vi "Listen.vi"() -> ()   [LabVIEW 2017]
uses:
  WebSocket.lvclass
panel:
  out "trimmed string":string
  out "element":string
  out "Headers":variant=variant("Accept-Encoding"=variant(string "gzip, deflate, br"), "Accept-Language"=variant(string "en-US,en;q=0.9"), "Cache-Control"=variant(string "no-cache"), "Connection"=variant(string "Upgrade"), "Host"=variant(string "localhost"), "Origin"=variant(string "http://tattsun.github.io"), "Pragma"=variant(string "no-cache"), "Sec-WebSocket-Extensions"=variant(string "permessage-deflate; client_max_window_bits"), "Sec-WebSocket-Key"=variant(string "dIZ2gIS4iTUMLhpa7t/LlA=="), "Sec-WebSocket-Version"=variant(string "13"), "Upgrade"=variant(string "websocket"), "User-Agent"=variant(string "Mozilla/5.0 (Windows NT 6.1; Win64; x64) AppleWebKit/537.36 (KHTML, like Gecko) Chrome/65.0.3325.181 Safari/537.36"))
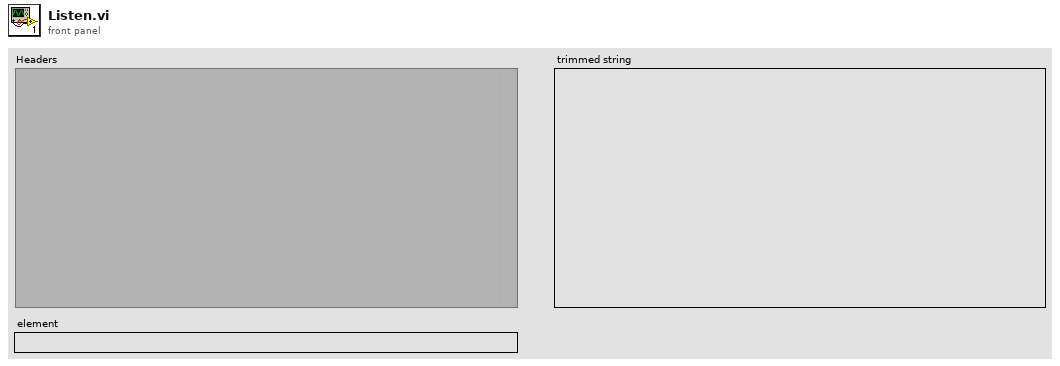
[diagram p1: front panel]
types:
  T1 = enum16{"Standard", "Buffered", "CRLF", "Immediate"}
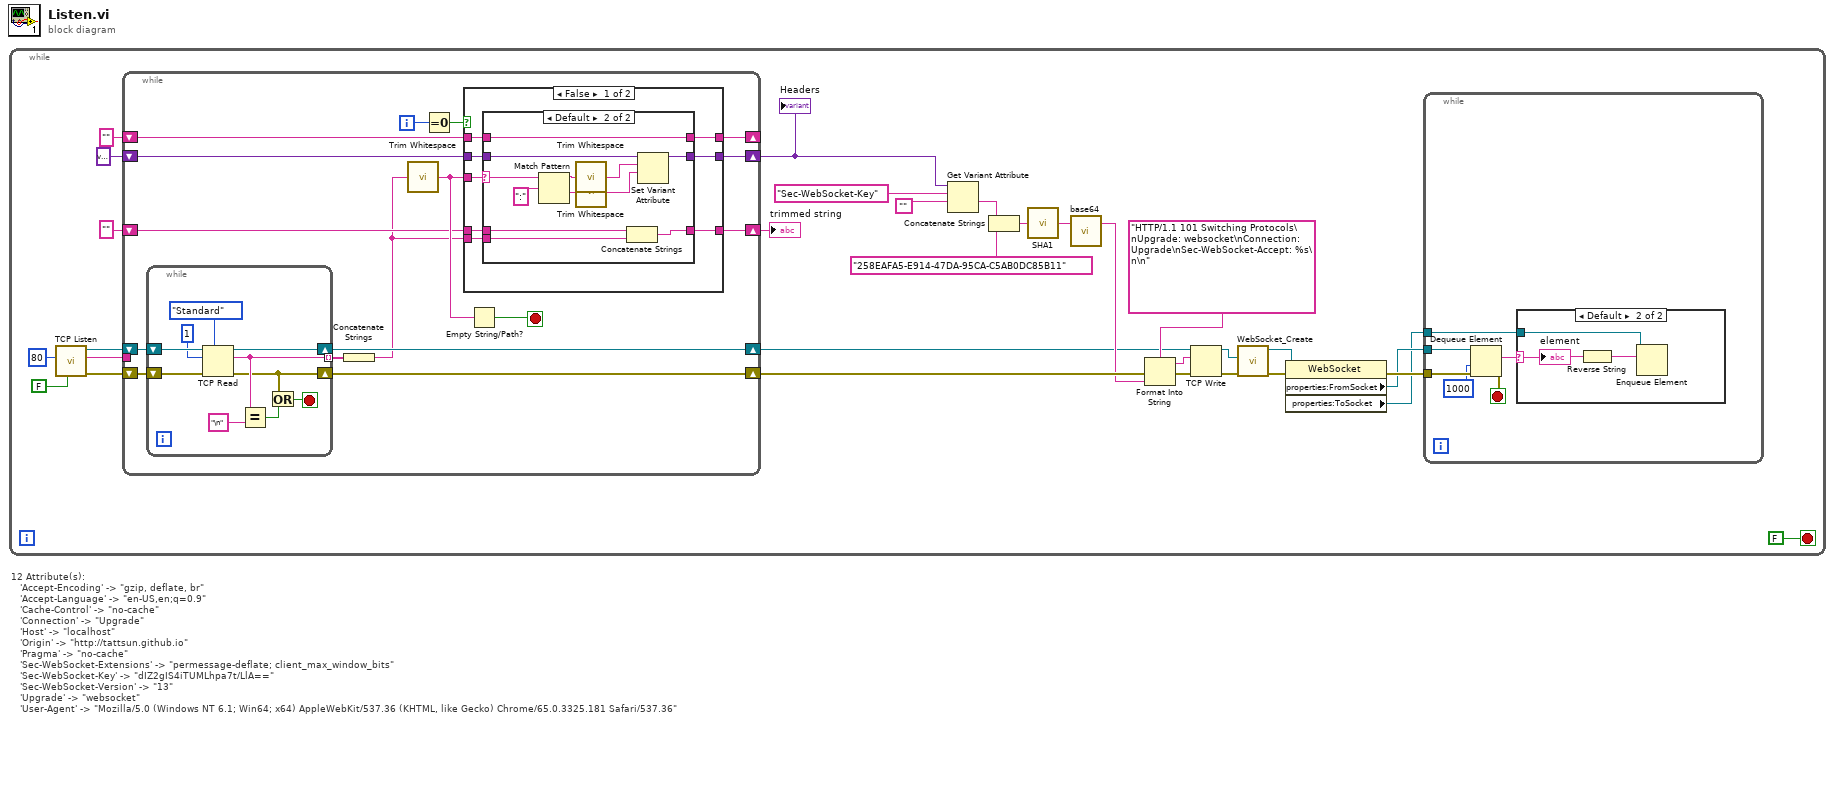
[diagram p0: block diagram]
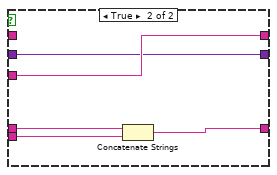
[diagram p4: hidden frame]
diagram:
  # "12 Attribute(s):\n   'Accept-Encoding' -> \"gzip, deflate, br\"\n   'Accept-Language' -> \"en-US,en;q=0.9\"\n   'Cache-Control' -> \"no-cache\"\n   'Connection' -> \"Upgrade\"\n   'Host' -> \"localhost\"\n   'Origin' -> \"http://tattsun.github.io\"\n   'Pragma' -> \"no-cache\"\n   'Sec-WebSocket-Extensions' -> \"permessage-deflate; client_max_window_bits\"\n   'Sec-WebSocket-Key' -> \"dIZ2gIS4iTUMLhpa7t/LlA==\"\n   'Sec-WebSocket-Version' -> \"13\"\n   'Upgrade' -> \"websocket\"\n   'User-Agent' -> \"Mozilla/5.0 (Windows NT 6.1; Win64; x64) AppleWebKit/537.36 (KHTML, like Gecko) Chrome/65.0.3325.181 Safari/537.36\""
  n1 = while {
    stop <- FALSE stop-if-true
    n2 = call <vilib>:"TCP Listen.vi"("resolve remote address (T)"=FALSE, "port"=u16 80) -> ("error out"=w27:errorcluster, "remote address"=w6:string, "connection ID"=w28:refnum<k5>)  [unwired: 5 in, 2 out]
    n3 = while {
      shift-right: [w46] -> w24
      shift-left: variant -> [w47]
      shift-right: [w51] -> _
      shift-left: "" ("trimmed string") -> [w50]
      shift-right: [w45] -> w13
      shift-left: w28 -> [w55]
      shift-right: [w44] -> w21
      shift-left: w27 -> [w54]
      shift-right: [w42] -> w8
      shift-left: "" ("trimmed string") -> [w41]
      tunnel: w6 -> [_]
      i -> [w53]
      stop <- w48 stop-if-true
      n4 = while {
        tunnel: [w60] -> w43 mode=indexing
        shift-right: [w61] -> w45
        shift-left: w55 -> [w65]
        shift-right: [w57] -> w44
        shift-left: w54 -> [w64]
        stop <- w56 stop-if-true
        n5 = TCP Read(connection ID=w65, bytes to read=1, error in (no error)=w64, 7:T1."Standard" ("mode (standard)")) -> (connection ID out=w61:refnum<k5>, data out=w60:string, error out=w57:errorcluster)  [unwired: 1 in]
        n6 = Equal?(x=w60, y="\n") -> (x = y?=w58:bool)
        n7 = Or(x=w57, y=w58) -> (x .or. y?=w56:bool)
      }
      n8 = Concatenate Strings(w43) -> (w40:string)
      n9 = call <vilib>:"Trim Whitespace.vi"("string"=w40) -> ("trimmed string"=w49:string)  [unwired: 1 in]
      n10 = Equal To 0?(x=w53) -> (x = 0?=w52:bool)
      n11 = case shown="False" w52 {
        tunnel: [w69 w93] -> w51
        tunnel: w49 -> [w71 w93]
        tunnel: w50 -> [w70 _]
        tunnel: w47 -> [w73 w92]
        tunnel: [w72 w92] -> w46
        tunnel: w40 -> [w68 w89]
        tunnel: [w67 w90] -> w42
        tunnel: w41 -> [w66 w91]
        frame False {
          n12 = case shown="Default" w71 {
            selector: w71 -> [_ w81]
            tunnel: w73 -> [w76 w85]
            tunnel: [w76 w84] -> w72
            tunnel: w70 -> [w75 w80]
            tunnel: [w75 w80] -> w69
            tunnel: w68 -> [_ w79]
            tunnel: [w74 w78] -> w67
            tunnel: w66 -> [w74 w77]
            frame "" {
            }
            frame Default {
              n13 = Match Pattern(string=w81, regular expression=":" ("trimmed string")) -> (before substring=w86:string, after substring=w87:string)  [unwired: 1 in, 2 out]
              n14 = call <vilib>:"Trim Whitespace.vi"("string"=w86) -> ("trimmed string"=w83:string)  [unwired: 1 in]
              n15 = call <vilib>:"Trim Whitespace.vi"("string"=w87) -> ("trimmed string"=w82:string)  [unwired: 1 in]
              n16 = Concatenate Strings(w77, w79) -> (w78:string)
              n17 = Set Variant Attribute(Variant=w85, name=w83, value=w82) -> (Variant out=w84:variant)  [unwired: 1 in, 2 out]
            }
          }
        }
        frame True {
          n18 = Concatenate Strings(w91, w89) -> (w90:string)
        }
      }
      n19 = Empty String/Path?(string/path=w49) -> (empty?=w48:bool)
    }
    "Headers" <- w24
    "trimmed string" <- w8
    n20 = Get Variant Attribute(Variant=w24, name="Sec-WebSocket-Key" ("trimmed string"), default value (empty Variant)="") -> (value=w20:string)  [unwired: 1 in, 3 out]
    n21 = Concatenate Strings(w20, "258EAFA5-E914-47DA-95CA-C5AB0DC85B11" ("trimmed string")) -> (w19:string)
    n22 = call "SHA1.vi"("String"=w19) -> ("SHA1"=w18:string)
    n23 = call "base64.vi"("string in"=w18) -> ("base64 out"=w17:string)  [unwired: 1 in, 1 out]
    n24 = Format Into String(format string="HTTP/1.1 101 Switching Protocols\nUpgrade: websocket\nConnection: Upgrade\nSec-WebSocket-Accept: %s\n\n" ("trimmed string"), error in=w21, w17) -> (resulting string=w14:string, error out=w15:errorcluster)  [unwired: 1 in]
    n25 = TCP Write(connection ID=w13, data in=w14, error in (no error)=w15) -> (connection ID out=w10:refnum<k5>, error out=w12:errorcluster)  [unwired: 1 in, 1 out]
    n26 = call "WebSocket_Create.vi"("error in (no error)"=w12, "Socket"=w10) -> ("error out"=w11:errorcluster, "reference out"=w4:refnum<class "WebSocket.lvclass">)  [unwired: 8 in]
    n27 = property class="WebSocket"(reference=w4, error in=w11) -> (error out=w5:errorcluster, "properties:FromSocket"=w3:refnum<queue>, "properties:ToSocket"=w2:refnum<queue>)  [unwired: 1 out]
    n28 = while {
      tunnel: w5 -> [w36]
      tunnel: w3 -> [w35]
      tunnel: w2 -> [w31]
      stop <- w34 stop-if-true
      n29 = Dequeue Element(queue=w35, timeout in ms (-1)=1000, error in (no error)=w36) -> (element=w32:string, error out=w34:errorcluster)  [unwired: 2 out]
      n30 = case shown="Default" w32 {
        selector: w32 -> [_ w38]
        tunnel: w31 -> [_ w39]
        frame "" {
        }
        frame Default {
          n31 = Reverse String(1:w38) -> (0:w37:string)
          n32 = Enqueue Element(queue=w39, element=w37) -> ()  [unwired: 2 in, 3 out]
          "element" <- w38
        }
      }
    }
  }
